vi "Increment Row TY720.vi"(5 "column":i32, 6 "Iteration":i32, 7 "row":i32, 8 "error in (no error)":errorcluster, 9 "Grandeza":string, 10 "NI_report in":refnum<class "NI_report.lvclass">, 11 "Ini File Output in":T1) -> (0 "error out":errorcluster, 2 "Last Row":i32, 3 "Ini File Output out":T1)   [LabVIEW 2015]
uses:
  controls/Ini File Output.ctl
  <vilib>/Utility/NIReport.llb/NI_report.lvclass
  <vilib>/addons/_office/NI_ReportGenerationToolkit.lvlib
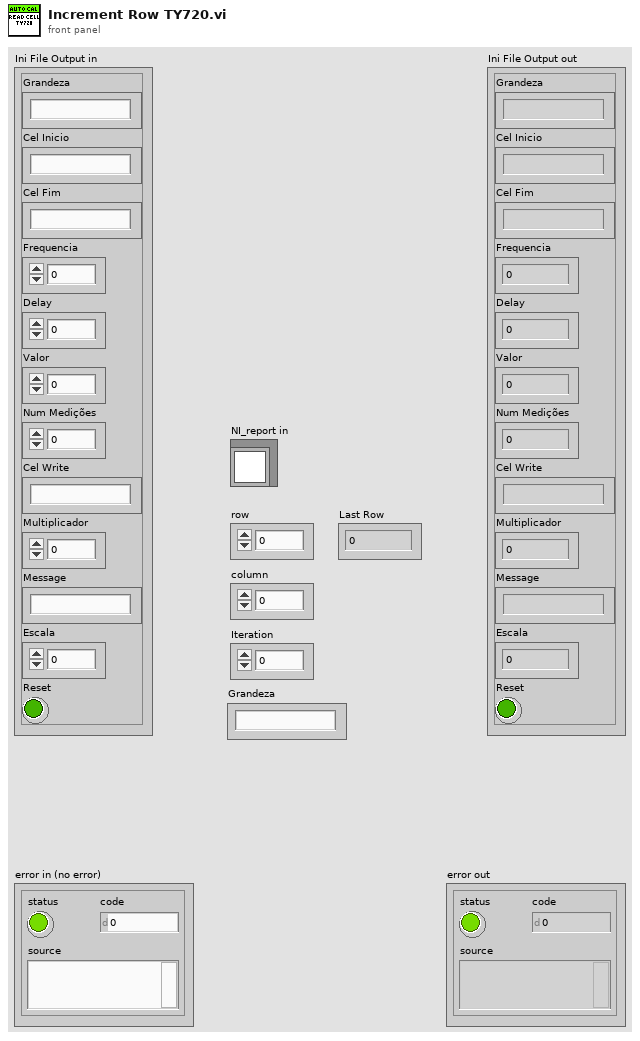
[diagram p1: front panel]
types:
  T1 = typedef "Ini File Output.ctl" = cluster{"Grandeza":string, "Cel Inicio":string, "Cel Fim":string, "Frequencia":dbl, "Delay":dbl, "Valor":dbl, "Num Medições":i32, "Cel Write":string, "Multiplicador":dbl, "Message":string, "Escala":dbl, "Reset":bool}
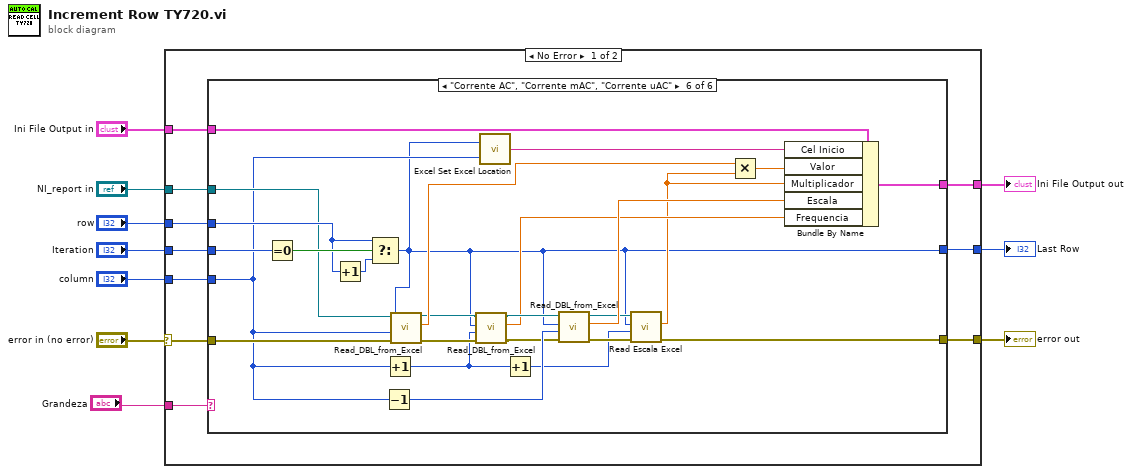
[diagram p0: block diagram]
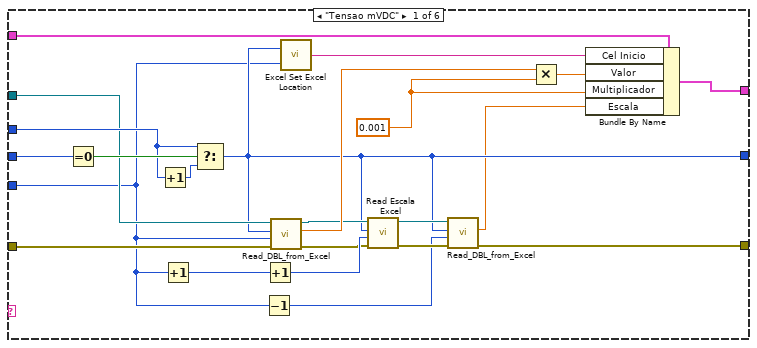
[diagram p2: hidden frame]
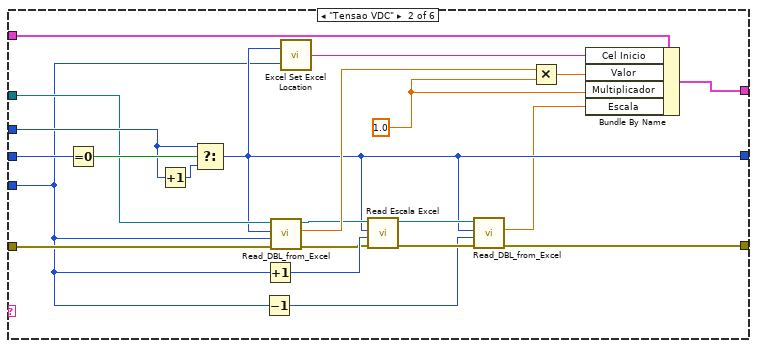
[diagram p3: hidden frame]
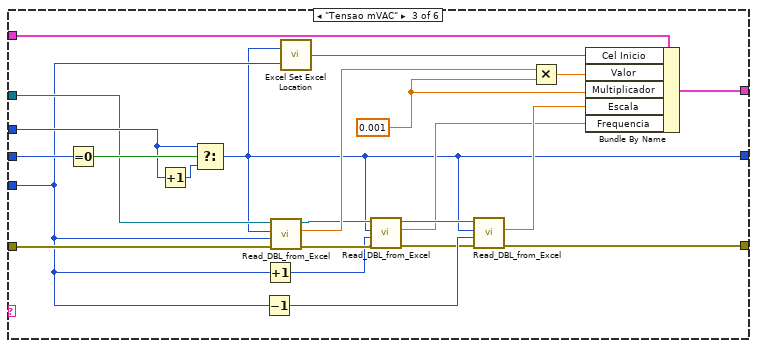
[diagram p4: hidden frame]
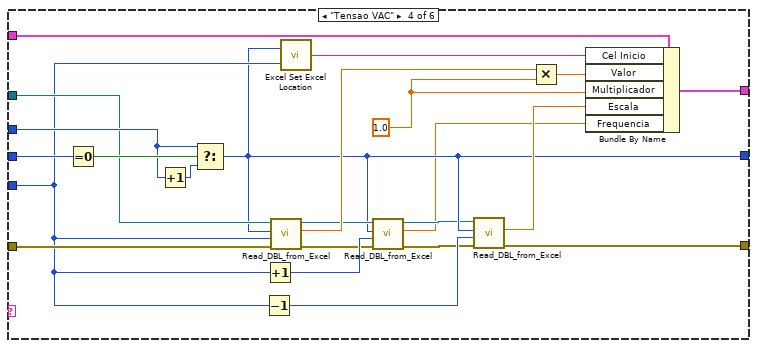
[diagram p5: hidden frame]
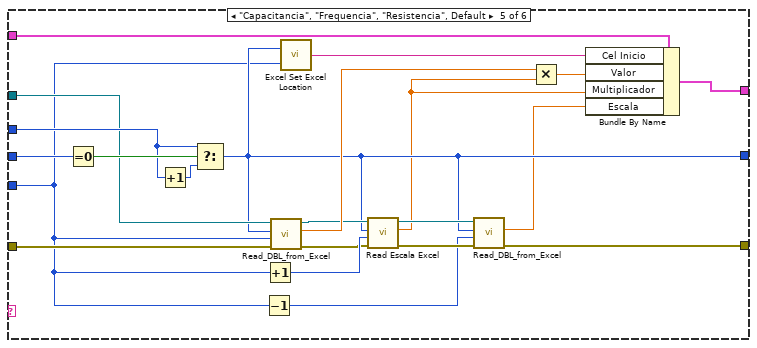
[diagram p6: hidden frame]
diagram:
  n1 = case shown="No Error" "error in (no error)" {
    selector: "error in (no error)" -> [w15 w160]
    tunnel: "column" -> [w13 _]
    tunnel: [w14 w161] -> w9
    tunnel: [w12 w160] -> w8
    tunnel: [w20 w162] -> w7
    tunnel: "Ini File Output in" -> [w19 w162]
    tunnel: "Iteration" -> [w18 _]
    tunnel: "row" -> [w17 w161]
    tunnel: "NI_report in" -> [w16 _]
    tunnel: "Grandeza" -> [w11 _]
    frame No Error {
      n2 = case shown="\"Corrente AC\", \"Corrente mAC\", \"Corrente uAC\"" w11 {
        tunnel: [w42 w64 w87 w110 w132 w158] -> w20
        tunnel: w19 -> [w41 w63 w73 w109 w131 w157]
        tunnel: w18 -> [w40 w62 w86 w108 w130 w156]
        tunnel: w17 -> [w37 w59 w83 w105 w127 w153]
        tunnel: w16 -> [w34 w56 w81 w103 w124 w151]
        tunnel: w15 -> [w33 w55 w80 w102 w123 w150]
        tunnel: [w27 w49 w67 w94 w117 w135] -> w14
        tunnel: w13 -> [w26 w48 w78 w100 w116 w148]
        tunnel: [w23 w46 w76 w98 w114 w137] -> w12
        frame "Tensao mVDC" {
          w21 = 0.001 ("y")
          n3 = Equal To 0?(x=w40) -> (x = 0?=w39:bool)
          n4 = Increment(x=w37) -> (x+1=w38:i32)
          n5 = Increment(x=w26) -> (x+1=w22:i32)
          n6 = Select(t=w37, s=w39, f=w38) -> (s? t:f=w27:i32)
          n7 = Decrement(x=w26) -> (x-1=w25:i32)
          n8 = Increment(x=w22) -> (x+1=w36:i32)
          n9 = call "Read_DBL_from_Excel.vi"("error in (no error)"=w33, "Colunm"=w26, "row"=w27, "NI_report in"=w34) -> ("error out"=w32:errorcluster, "data"=w31:dbl, "NI_report Out"=w30:refnum<class "NI_report.lvclass">)  [unwired: 5 in]
          n10 = call <vilib>:"Excel Set Excel Location.vi"("column"=w26, "row"=w27) -> ("cell's name"=w43:string)
          n11 = call "Read Escala Excel.vi"("error in (no error)"=w32, "Colunm"=w36, "row"=w27, "NI_report in"=w30) -> ("error out"=w28:errorcluster, "NI_report Out"=w29:refnum<class "NI_report.lvclass">)  [unwired: 5 in, 1 out]
          n12 = call "Read_DBL_from_Excel.vi"("error in (no error)"=w28, "Colunm"=w25, "row"=w27, "NI_report in"=w29) -> ("error out"=w23:errorcluster, "data"=w24:dbl)  [unwired: 5 in, 1 out]
          n13 = Multiply(x=w31, y=w21) -> (x*y=w35:dbl)
          n14 = Bundle By Name(cluster=w41, "Cel Inicio"=w43, "Valor"=w35, "Multiplicador"=w21, "Escala"=w24) -> (w42:T1)
        }
        frame "Tensao VDC" {
          w45 = 1.0 ("y")
          n15 = Equal To 0?(x=w62) -> (x = 0?=w61:bool)
          n16 = Increment(x=w59) -> (x+1=w60:i32)
          n17 = Select(t=w59, s=w61, f=w60) -> (s? t:f=w49:i32)
          n18 = Decrement(x=w48) -> (x-1=w47:i32)
          n19 = Increment(x=w48) -> (x+1=w58:i32)
          n20 = call "Read_DBL_from_Excel.vi"("error in (no error)"=w55, "Colunm"=w48, "row"=w49, "NI_report in"=w56) -> ("error out"=w54:errorcluster, "data"=w53:dbl, "NI_report Out"=w52:refnum<class "NI_report.lvclass">)  [unwired: 5 in]
          n21 = call <vilib>:"Excel Set Excel Location.vi"("column"=w48, "row"=w49) -> ("cell's name"=w65:string)
          n22 = call "Read Escala Excel.vi"("error in (no error)"=w54, "Colunm"=w58, "row"=w49, "NI_report in"=w52) -> ("error out"=w50:errorcluster, "NI_report Out"=w51:refnum<class "NI_report.lvclass">)  [unwired: 5 in, 1 out]
          n23 = call "Read_DBL_from_Excel.vi"("error in (no error)"=w50, "Colunm"=w47, "row"=w49, "NI_report in"=w51) -> ("error out"=w46:errorcluster, "data"=w44:dbl)  [unwired: 5 in, 1 out]
          n24 = Multiply(x=w53, y=w45) -> (x*y=w57:dbl)
          n25 = Bundle By Name(cluster=w63, "Cel Inicio"=w65, "Valor"=w57, "Multiplicador"=w45, "Escala"=w44) -> (w64:T1)
        }
        frame "Tensao mVAC" {
          w75 = 0.001 ("y")
          n26 = Equal To 0?(x=w86) -> (x = 0?=w85:bool)
          n27 = Increment(x=w83) -> (x+1=w84:i32)
          n28 = Select(t=w83, s=w85, f=w84) -> (s? t:f=w67:i32)
          n29 = Decrement(x=w78) -> (x-1=w77:i32)
          n30 = Increment(x=w78) -> (x+1=w66:i32)
          n31 = call "Read_DBL_from_Excel.vi"("error in (no error)"=w80, "Colunm"=w78, "row"=w67, "NI_report in"=w81) -> ("error out"=w71:errorcluster, "data"=w79:dbl, "NI_report Out"=w72:refnum<class "NI_report.lvclass">)  [unwired: 5 in]
          n32 = call <vilib>:"Excel Set Excel Location.vi"("column"=w78, "row"=w67) -> ("cell's name"=w88:string)
          n33 = call "Read_DBL_from_Excel.vi"("error in (no error)"=w71, "Colunm"=w66, "row"=w67, "NI_report in"=w72) -> ("error out"=w70:errorcluster, "data"=w68:dbl, "NI_report Out"=w69:refnum<class "NI_report.lvclass">)  [unwired: 5 in]
          n34 = call "Read_DBL_from_Excel.vi"("error in (no error)"=w70, "Colunm"=w77, "row"=w67, "NI_report in"=w69) -> ("error out"=w76:errorcluster, "data"=w74:dbl)  [unwired: 5 in, 1 out]
          n35 = Multiply(x=w79, y=w75) -> (x*y=w82:dbl)
          n36 = Bundle By Name(cluster=w73, "Cel Inicio"=w88, "Valor"=w82, "Multiplicador"=w75, "Escala"=w74, "Frequencia"=w68) -> (w87:T1)
        }
        frame "Tensao VAC" {
          w97 = 1.0 ("y")
          n37 = Equal To 0?(x=w108) -> (x = 0?=w107:bool)
          n38 = Increment(x=w105) -> (x+1=w106:i32)
          n39 = Select(t=w105, s=w107, f=w106) -> (s? t:f=w94:i32)
          n40 = Decrement(x=w100) -> (x-1=w99:i32)
          n41 = Increment(x=w100) -> (x+1=w90:i32)
          n42 = call "Read_DBL_from_Excel.vi"("error in (no error)"=w102, "Colunm"=w100, "row"=w94, "NI_report in"=w103) -> ("error out"=w89:errorcluster, "data"=w101:dbl, "NI_report Out"=w95:refnum<class "NI_report.lvclass">)  [unwired: 5 in]
          n43 = call <vilib>:"Excel Set Excel Location.vi"("column"=w100, "row"=w94) -> ("cell's name"=w111:string)
          n44 = call "Read_DBL_from_Excel.vi"("error in (no error)"=w89, "Colunm"=w90, "row"=w94, "NI_report in"=w95) -> ("error out"=w92:errorcluster, "data"=w91:dbl, "NI_report Out"=w93:refnum<class "NI_report.lvclass">)  [unwired: 5 in]
          n45 = call "Read_DBL_from_Excel.vi"("error in (no error)"=w92, "Colunm"=w99, "row"=w94, "NI_report in"=w93) -> ("error out"=w98:errorcluster, "data"=w96:dbl)  [unwired: 5 in, 1 out]
          n46 = Multiply(x=w101, y=w97) -> (x*y=w104:dbl)
          n47 = Bundle By Name(cluster=w109, "Cel Inicio"=w111, "Valor"=w104, "Multiplicador"=w97, "Escala"=w96, "Frequencia"=w91) -> (w110:T1)
        }
        frame "Capacitancia", "Frequencia", "Resistencia", Default {
          n48 = Equal To 0?(x=w130) -> (x = 0?=w129:bool)
          n49 = Increment(x=w127) -> (x+1=w128:i32)
          n50 = Select(t=w127, s=w129, f=w128) -> (s? t:f=w117:i32)
          n51 = Decrement(x=w116) -> (x-1=w115:i32)
          n52 = Increment(x=w116) -> (x+1=w126:i32)
          n53 = call "Read_DBL_from_Excel.vi"("error in (no error)"=w123, "Colunm"=w116, "row"=w117, "NI_report in"=w124) -> ("error out"=w122:errorcluster, "data"=w121:dbl, "NI_report Out"=w120:refnum<class "NI_report.lvclass">)  [unwired: 5 in]
          n54 = call <vilib>:"Excel Set Excel Location.vi"("column"=w116, "row"=w117) -> ("cell's name"=w133:string)
          n55 = call "Read Escala Excel.vi"("error in (no error)"=w122, "Colunm"=w126, "row"=w117, "NI_report in"=w120) -> ("error out"=w118:errorcluster, "data"=w112:dbl, "NI_report Out"=w119:refnum<class "NI_report.lvclass">)  [unwired: 5 in]
          n56 = call "Read_DBL_from_Excel.vi"("error in (no error)"=w118, "Colunm"=w115, "row"=w117, "NI_report in"=w119) -> ("error out"=w114:errorcluster, "data"=w113:dbl)  [unwired: 5 in, 1 out]
          n57 = Multiply(x=w121, y=w112) -> (x*y=w125:dbl)
          n58 = Bundle By Name(cluster=w131, "Cel Inicio"=w133, "Valor"=w125, "Multiplicador"=w112, "Escala"=w113) -> (w132:T1)
        }
        frame "Corrente AC", "Corrente mAC", "Corrente uAC" {
          n59 = Equal To 0?(x=w156) -> (x = 0?=w155:bool)
          n60 = Increment(x=w153) -> (x+1=w154:i32)
          n61 = Select(t=w153, s=w155, f=w154) -> (s? t:f=w135:i32)
          n62 = Decrement(x=w148) -> (x-1=w147:i32)
          n63 = Increment(x=w148) -> (x+1=w140:i32)
          n64 = call "Read_DBL_from_Excel.vi"("error in (no error)"=w150, "Colunm"=w148, "row"=w135, "NI_report in"=w151) -> ("error out"=w141:errorcluster, "data"=w149:dbl, "NI_report Out"=w145:refnum<class "NI_report.lvclass">)  [unwired: 5 in]
          n65 = call "Read_DBL_from_Excel.vi"("error in (no error)"=w141, "Colunm"=w140, "row"=w135, "NI_report in"=w145) -> ("error out"=w142:errorcluster, "data"=w143:dbl, "NI_report Out"=w144:refnum<class "NI_report.lvclass">)  [unwired: 5 in]
          n66 = call <vilib>:"Excel Set Excel Location.vi"("column"=w148, "row"=w135) -> ("cell's name"=w159:string)
          n67 = Increment(x=w140) -> (x+1=w134:i32)
          n68 = call "Read_DBL_from_Excel.vi"("error in (no error)"=w142, "Colunm"=w147, "row"=w135, "NI_report in"=w144) -> ("error out"=w136:errorcluster, "data"=w146:dbl, "NI_report Out"=w139:refnum<class "NI_report.lvclass">)  [unwired: 5 in]
          n69 = call "Read Escala Excel.vi"("error in (no error)"=w136, "Colunm"=w134, "row"=w135, "NI_report in"=w139) -> ("error out"=w137:errorcluster, "data"=w138:dbl)  [unwired: 5 in, 1 out]
          n70 = Multiply(x=w149, y=w138) -> (x*y=w152:dbl)
          n71 = Bundle By Name(cluster=w157, "Cel Inicio"=w159, "Valor"=w152, "Multiplicador"=w138, "Escala"=w146, "Frequencia"=w143) -> (w158:T1)
        }
      }
    }
    frame Error {
    }
  }
  "Last Row" <- w9
  "error out" <- w8
  "Ini File Output out" <- w7
